vi "6229 Write_Rev1.vi"(0 "Arbitrary Waveform\nArray of Channels":T1(array[cluster])=[[{"AC Frequency (kHz)"=0.0, " Initial AC Ampl. (p-p/2)"=0.0, "Final AC Ampl."=0.0, "Initial DC Value"=7.0, "Final DC Value"=1.0, "Constant/Tau"=2.0, "Gamma AC"=1.0, "String"="Channel 0 A", "Gamma DC/Beta"=1.0}, {"AC Frequency (kHz)"=40.0, " Initial AC Ampl. (p-p/2)"=0.0, "Final AC Ampl."=0.0, "Initial DC Value"=1.0, "Final DC Value"=1.0, "Constant/Tau"=2.0, "Gamma AC"=1.0, "String"="Channel 0 B", "Gamma DC/Beta"=1.0}, {"AC Frequency (kHz)"=40.0, " Initial AC Ampl. (p-p/2)"=0.0, "Final AC Ampl."=0.0, "Initial DC Value"=1.0, "Final DC Value"=1.0, "Constant/Tau"=2.0, "Gamma AC"=1.0, "String"="Channel 0 C", "Gamma DC/Beta"=1.0}, {"AC Frequency (kHz)"=0.0, " Initial AC Ampl. (p-p/2)"=0.0, "Final AC Ampl."=0.0, "Initial DC Value"=1.0, "Final DC Value"=7.0, "Constant/Tau"=2.0, "Gamma AC"=0.0, "String"="Channel 0 D", "Gamma DC/Beta"=1.0}, {"AC Frequency (kHz)"=0.0, " Initial AC Ampl. (p-p/2)"=0.0, "Final AC Ampl."=0.0, "Initial DC Value"=7.0, "Final DC Value"=6.0, "Constant/Tau"=2.0, "Gamma AC"=0.0, "String"="Channel 0 E", "Gamma DC/Beta"=1.0}], [{"AC Frequency (kHz)"=10.0, " Initial AC Ampl. (p-p/2)"=5.0, "Final AC Ampl."=0.0, "Initial DC Value"=0.2, "Final DC Value"=0.16, "Constant/Tau"=0.25, "Gamma AC"=1.0, "String"="Channel 1 A", "Gamma DC/Beta"=1.0}, {"AC Frequency (kHz)"=10.0, " Initial AC Ampl. (p-p/2)"=5.0, "Final AC Ampl."=0.0, "Initial DC Value"=0.16, "Final DC Value"=0.16, "Constant/Tau"=0.25, "Gamma AC"=1.0, "String"="Channel 1 B", "Gamma DC/Beta"=1.0}, {"AC Frequency (kHz)"=10.0, " Initial AC Ampl. (p-p/2)"=0.0, "Final AC Ampl."=0.0, "Initial DC Value"=0.0, "Final DC Value"=0.0, "Constant/Tau"=0.25, "Gamma AC"=1.0, "String"="Channel 1 C", "Gamma DC/Beta"=1.0}, {"AC Frequency (kHz)"=0.0, " Initial AC Ampl. (p-p/2)"=0.0, "Final AC Ampl."=0.0, "Initial DC Value"=1.0, "Final DC Value"=1.0, "Constant/Tau"=199.2, "Gamma AC"=0.0, "String"="Channel 1 D", "Gamma DC/Beta"=1.0}, {"AC Frequency (kHz)"=0.0, " Initial AC Ampl. (p-p/2)"=0.0, "Final AC Ampl."=0.0, "Initial DC Value"=1.0, "Final DC Value"=1.0, "Constant/Tau"=199.2, "Gamma AC"=0.0, "String"="Channel 1 E", "Gamma DC/Beta"=1.0}], [{"AC Frequency (kHz)"=10.0, " Initial AC Ampl. (p-p/2)"=0.0, "Final AC Ampl."=0.0, "Initial DC Value"=0.007, "Final DC Value"=0.06, "Constant/Tau"=0.0, "Gamma AC"=1.0, "String"="Channel 2 A", "Gamma DC/Beta"=1.0}, {"AC Frequency (kHz)"=10.0, " Initial AC Ampl. (p-p/2)"=0.0, "Final AC Ampl."=0.0, "Initial DC Value"=0.06, "Final DC Value"=0.06, "Constant/Tau"=0.0, "Gamma AC"=1.0, "String"="Channel 2 B", "Gamma DC/Beta"=1.0}, {"AC Frequency (kHz)"=10.0, " Initial AC Ampl. (p-p/2)"=0.0, "Final AC Ampl."=0.0, "Initial DC Value"=0.0, "Final DC Value"=0.0, "Constant/Tau"=0.0, "Gamma AC"=1.0, "String"="Channel 2 C", "Gamma DC/Beta"=1.0}, {"AC Frequency (kHz)"=0.0, " Initial AC Ampl. (p-p/2)"=0.0, "Final AC Ampl."=0.0, "Initial DC Value"=1.0, "Final DC Value"=1.0, "Constant/Tau"=199.2, "Gamma AC"=0.0, "String"="", "Gamma DC/Beta"=1.0}, {"AC Frequency (kHz)"=0.0, " Initial AC Ampl. (p-p/2)"=0.0, "Final AC Ampl."=0.0, "Initial DC Value"=1.0, "Final DC Value"=1.0, "Constant/Tau"=199.2, "Gamma AC"=0.0, "String"="", "Gamma DC/Beta"=1.0}], [{"AC Frequency (kHz)"=10.0, " Initial AC Ampl. (p-p/2)"=0.0, "Final AC Ampl."=0.0, "Initial DC Value"=1.0, "Final DC Value"=1.0, "Constant/Tau"=199.2, "Gamma AC"=1.0, "String"="Channel 3 A", "Gamma DC/Beta"=1.0}, {"AC Frequency (kHz)"=10.0, " Initial AC Ampl. (p-p/2)"=0.0, "Final AC Ampl."=0.0, "Initial DC Value"=1.0, "Final DC Value"=1.0, "Constant/Tau"=199.2, "Gamma AC"=1.0, "String"="Channel 3 B", "Gamma DC/Beta"=1.0}, {"AC Frequency (kHz)"=10.0, " Initial AC Ampl. (p-p/2)"=0.0, "Final AC Ampl."=0.0, "Initial DC Value"=1.0, "Final DC Value"=1.0, "Constant/Tau"=199.2, "Gamma AC"=1.0, "String"="Channel 3 C", "Gamma DC/Beta"=1.0}, {"AC Frequency (kHz)"=0.0, " Initial AC Ampl. (p-p/2)"=0.0, "Final AC Ampl."=0.0, "Initial DC Value"=1.0, "Final DC Value"=1.0, "Constant/Tau"=199.2, "Gamma AC"=0.0, "String"="", "Gamma DC/Beta"=1.0}, {"AC Frequency (kHz)"=0.0, " Initial AC Ampl. (p-p/2)"=0.0, "Final AC Ampl."=0.0, "Initial DC Value"=1.0, "Final DC Value"=1.0, "Constant/Tau"=199.2, "Gamma AC"=0.0, "String"="", "Gamma DC/Beta"=1.0}], [{"AC Frequency (kHz)"=10.0, " Initial AC Ampl. (p-p/2)"=0.0, "Final AC Ampl."=0.0, "Initial DC Value"=-0.1, "Final DC Value"=-0.04, "Constant/Tau"=199.2, "Gamma AC"=1.0, "String"="Channel 4 A", "Gamma DC/Beta"=1.0}, {"AC Frequency (kHz)"=10.0, " Initial AC Ampl. (p-p/2)"=0.0, "Final AC Ampl."=0.0, "Initial DC Value"=-0.1, "Final DC Value"=-0.04, "Constant/Tau"=199.2, "Gamma AC"=1.0, "String"="Channel 4 B", "Gamma DC/Beta"=1.0}, {"AC Frequency (kHz)"=10.0, " Initial AC Ampl. (p-p/2)"=0.0, "Final AC Ampl."=0.0, "Initial DC Value"=-0.1, "Final DC Value"=-0.04, "Constant/Tau"=199.2, "Gamma AC"=1.0, "String"="Channel 4 C", "Gamma DC/Beta"=1.0}, {"AC Frequency (kHz)"=0.0, " Initial AC Ampl. (p-p/2)"=0.0, "Final AC Ampl."=0.0, "Initial DC Value"=1.0, "Final DC Value"=1.0, "Constant/Tau"=199.2, "Gamma AC"=0.0, "String"="", "Gamma DC/Beta"=1.0}, {"AC Frequency (kHz)"=0.0, " Initial AC Ampl. (p-p/2)"=0.0, "Final AC Ampl."=0.0, "Initial DC Value"=1.0, "Final DC Value"=1.0, "Constant/Tau"=199.2, "Gamma AC"=0.0, "String"="", "Gamma DC/Beta"=1.0}], [{"AC Frequency (kHz)"=10.0, " Initial AC Ampl. (p-p/2)"=0.0, "Final AC Ampl."=0.0, "Initial DC Value"=-0.1, "Final DC Value"=-0.04, "Constant/Tau"=199.2, "Gamma AC"=1.0, "String"="Channel 5 A", "Gamma DC/Beta"=1.0}, {"AC Frequency (kHz)"=10.0, " Initial AC Ampl. (p-p/2)"=0.0, "Final AC Ampl."=0.0, "Initial DC Value"=-0.1, "Final DC Value"=-0.04, "Constant/Tau"=199.2, "Gamma AC"=1.0, "String"="Channel 5 B", "Gamma DC/Beta"=1.0}, {"AC Frequency (kHz)"=10.0, " Initial AC Ampl. (p-p/2)"=0.0, "Final AC Ampl."=0.0, "Initial DC Value"=-0.1, "Final DC Value"=-0.04, "Constant/Tau"=199.2, "Gamma AC"=1.0, "String"="Channel 5 C", "Gamma DC/Beta"=1.0}, {"AC Frequency (kHz)"=0.0, " Initial AC Ampl. (p-p/2)"=0.0, "Final AC Ampl."=0.0, "Initial DC Value"=1.0, "Final DC Value"=1.0, "Constant/Tau"=199.2, "Gamma AC"=0.0, "String"="", "Gamma DC/Beta"=1.0}, {"AC Frequency (kHz)"=0.0, " Initial AC Ampl. (p-p/2)"=0.0, "Final AC Ampl."=0.0, "Initial DC Value"=1.0, "Final DC Value"=1.0, "Constant/Tau"=199.2, "Gamma AC"=0.0, "String"="", "Gamma DC/Beta"=1.0}], [{"AC Frequency (kHz)"=10.0, " Initial AC Ampl. (p-p/2)"=0.0, "Final AC Ampl."=0.0, "Initial DC Value"=-0.1, "Final DC Value"=-0.04, "Constant/Tau"=199.2, "Gamma AC"=1.0, "String"="Channel 6 A", "Gamma DC/Beta"=1.0}, {"AC Frequency (kHz)"=10.0, " Initial AC Ampl. (p-p/2)"=0.0, "Final AC Ampl."=0.0, "Initial DC Value"=-0.1, "Final DC Value"=-0.04, "Constant/Tau"=199.2, "Gamma AC"=1.0, "String"="Channel 6 B", "Gamma DC/Beta"=1.0}, {"AC Frequency (kHz)"=10.0, " Initial AC Ampl. (p-p/2)"=0.0, "Final AC Ampl."=0.0, "Initial DC Value"=-0.1, "Final DC Value"=-0.04, "Constant/Tau"=199.2, "Gamma AC"=1.0, "String"="Channel 6 C", "Gamma DC/Beta"=1.0}, {"AC Frequency (kHz)"=0.0, " Initial AC Ampl. (p-p/2)"=0.0, "Final AC Ampl."=0.0, "Initial DC Value"=1.0, "Final DC Value"=1.0, "Constant/Tau"=199.2, "Gamma AC"=0.0, "String"="", "Gamma DC/Beta"=1.0}, {"AC Frequency (kHz)"=0.0, " Initial AC Ampl. (p-p/2)"=0.0, "Final AC Ampl."=0.0, "Initial DC Value"=1.0, "Final DC Value"=1.0, "Constant/Tau"=199.2, "Gamma AC"=0.0, "String"="", "Gamma DC/Beta"=1.0}], [{"AC Frequency (kHz)"=10.0, " Initial AC Ampl. (p-p/2)"=0.0, "Final AC Ampl."=0.0, "Initial DC Value"=-0.1, "Final DC Value"=-0.04, "Constant/Tau"=199.2, "Gamma AC"=1.0, "String"="Channel 7 A", "Gamma DC/Beta"=1.0}, {"AC Frequency (kHz)"=10.0, " Initial AC Ampl. (p-p/2)"=0.0, "Final AC Ampl."=0.0, "Initial DC Value"=-0.1, "Final DC Value"=-0.04, "Constant/Tau"=199.2, "Gamma AC"=1.0, "String"="Channel 7 B", "Gamma DC/Beta"=1.0}, {"AC Frequency (kHz)"=10.0, " Initial AC Ampl. (p-p/2)"=0.0, "Final AC Ampl."=0.0, "Initial DC Value"=-0.1, "Final DC Value"=-0.04, "Constant/Tau"=199.2, "Gamma AC"=1.0, "String"="Channel 7 C", "Gamma DC/Beta"=1.0}, {"AC Frequency (kHz)"=0.0, " Initial AC Ampl. (p-p/2)"=0.0, "Final AC Ampl."=0.0, "Initial DC Value"=1.0, "Final DC Value"=1.0, "Constant/Tau"=199.2, "Gamma AC"=0.0, "String"="", "Gamma DC/Beta"=1.0}, {"AC Frequency (kHz)"=0.0, " Initial AC Ampl. (p-p/2)"=0.0, "Final AC Ampl."=0.0, "Initial DC Value"=1.0, "Final DC Value"=1.0, "Constant/Tau"=199.2, "Gamma AC"=0.0, "String"="", "Gamma DC/Beta"=1.0}]] {"Gamma DC/Beta" format="%.2f"; "Gamma AC" format="%.2f"; "Constant/Tau" min=0.0 max=240.0 format="%.4f"; "Final DC Value" format="%.3f"; "Initial DC Value" format="%.3f"; "Final AC Ampl." format="%.3f"; "Initial AC Ampl. (p-p/2)" format="%.3f"; "AC Frequency (kHz)" format="%.2f"}, 2 "Channel to plot":i32 min=0 max=7, 3 "Unit Conversions":u16[](array[ring])=[0, 0, 2, 3, 4, 0, 0, 0] items=["Volts-to-Volts Power Law", "Evaporation Formula", "Dimple Evaporation"], 4 "Interval Lengths (ms)":dbl[](array[numeric])=[120.0, 16.0, 484.0, 700.0, 100.0] format="%.3f", 5 "Channel Controls":bool[](array[boolean])=[TRUE, TRUE, FALSE, FALSE, FALSE, FALSE, FALSE, FALSE], 6 "ON or OFF?":bool[](array[boolean])=[TRUE, TRUE, TRUE, FALSE, FALSE], 11 "error in":errorcluster, 12 "Dither Control":u16(ring)=1 items=["Disable Dither", "Enable Dither"]) -> (9 "Sampling Rate":dbl=2882.3529411764707 format="%.2f", 10 "= Total Waveform\nTime (ms)":dbl=1420.0 format="%.3f", 13 "Waveform on Channel to Plot":cluster{dbl[], dbl[]}(graph), 14 "signal out":waveform(dbl)[](graph)=[{"t0"=timestamp(0 s since 1904-01-01), "dt"=0.00034693877551020405, "Y"=array[4091 elements]}, {"t0"=timestamp(0 s since 1904-01-01), "dt"=0.00034693877551020405, "Y"=array[4091 elements]}], 15 "error out":errorcluster)   [LabVIEW 2013]
uses:
  <vilib>/Utility/error.llb/DialogType.ctl
  <vilib>/DAQmx/write.llb/DAQmx Write (Analog 1D Wfm NChan NSamp).vi
  <vilib>/DAQmx/configure/timing.llb/DAQmx Timing (Sample Clock).vi
  <vilib>/DAQmx/create/channels.llb/DAQmx Create Channel (CO-Pulse Generation-Frequency).vi
  <vilib>/DAQmx/configure/timing.llb/DAQmx Timing (Implicit).vi
  <vilib>/DAQmx/configure/trigger.llb/DAQmx Start Trigger (Digital Edge).vi
  <vilib>/DAQmx/miscellaneous.llb/DAQmx Fill In Error Info.vi
  <resource>/objmgr/daqmx.rc
panel:
  in  "Case Constant\n(See Context Help) 3":bool=TRUE
  in  "Case Constant\n(See Context Help) 2":bool
  in  "Dither Control":u16
  in  "Case Constant\n(See Context Help)":bool
  in  "Dither Control":u16
  out "number of samples written per channel":u32
  out "Pmod Graph":dbl[][](graph)
  out "wvfrm size":i32=4091
  out "x+y 2":dbl=1.42
  out "Numeric":i32=287
  out "6229 counter task out":refnum<k21>="Counter Output"
  out "6229 lattice loading task out":refnum<k21>="Adiabatic Loading"
  out "Array":dbl[][](array[numeric])
  out "6229 Status":string="PCI-6221 OK"
  out "total points":dbl=4092.0 format="%.2f"
  out "Points per Segment":dbl[](array[numeric])=[345.0, 46.0, 1395.0, 2017.0, 288.0] format="%.2f"
  # "Warning! Constant for interval A does not set all intervals for 86 Sr frequency"
  # "Controls"
  # "Volts to Volts Power Law Formula\nf100=DCinitial +(DCfinal-DCinitial)*(time/intervaltime)**gammaDC;"
  # "Don't change"
  # "Note: B-field to Voltage\nConversion not yet\nimplemented.  Must \ninsert appropriate\nformulae."
  # "CH 0"
  # "CH 1"
  # "CH 2"
  # "CH 3"
  # "Evaporation Formula\nf100=Initial/((1+(time/tau))**beta)+Final;"
  # "Initial DC = U1, Constant = Tau\nGamma DC = Beta"
  # "Interval A"
  # "Interval B"
  # "Interval C"
  # "Interval D"
  # "Interval E"
  # "Interval F"
  # "Output"
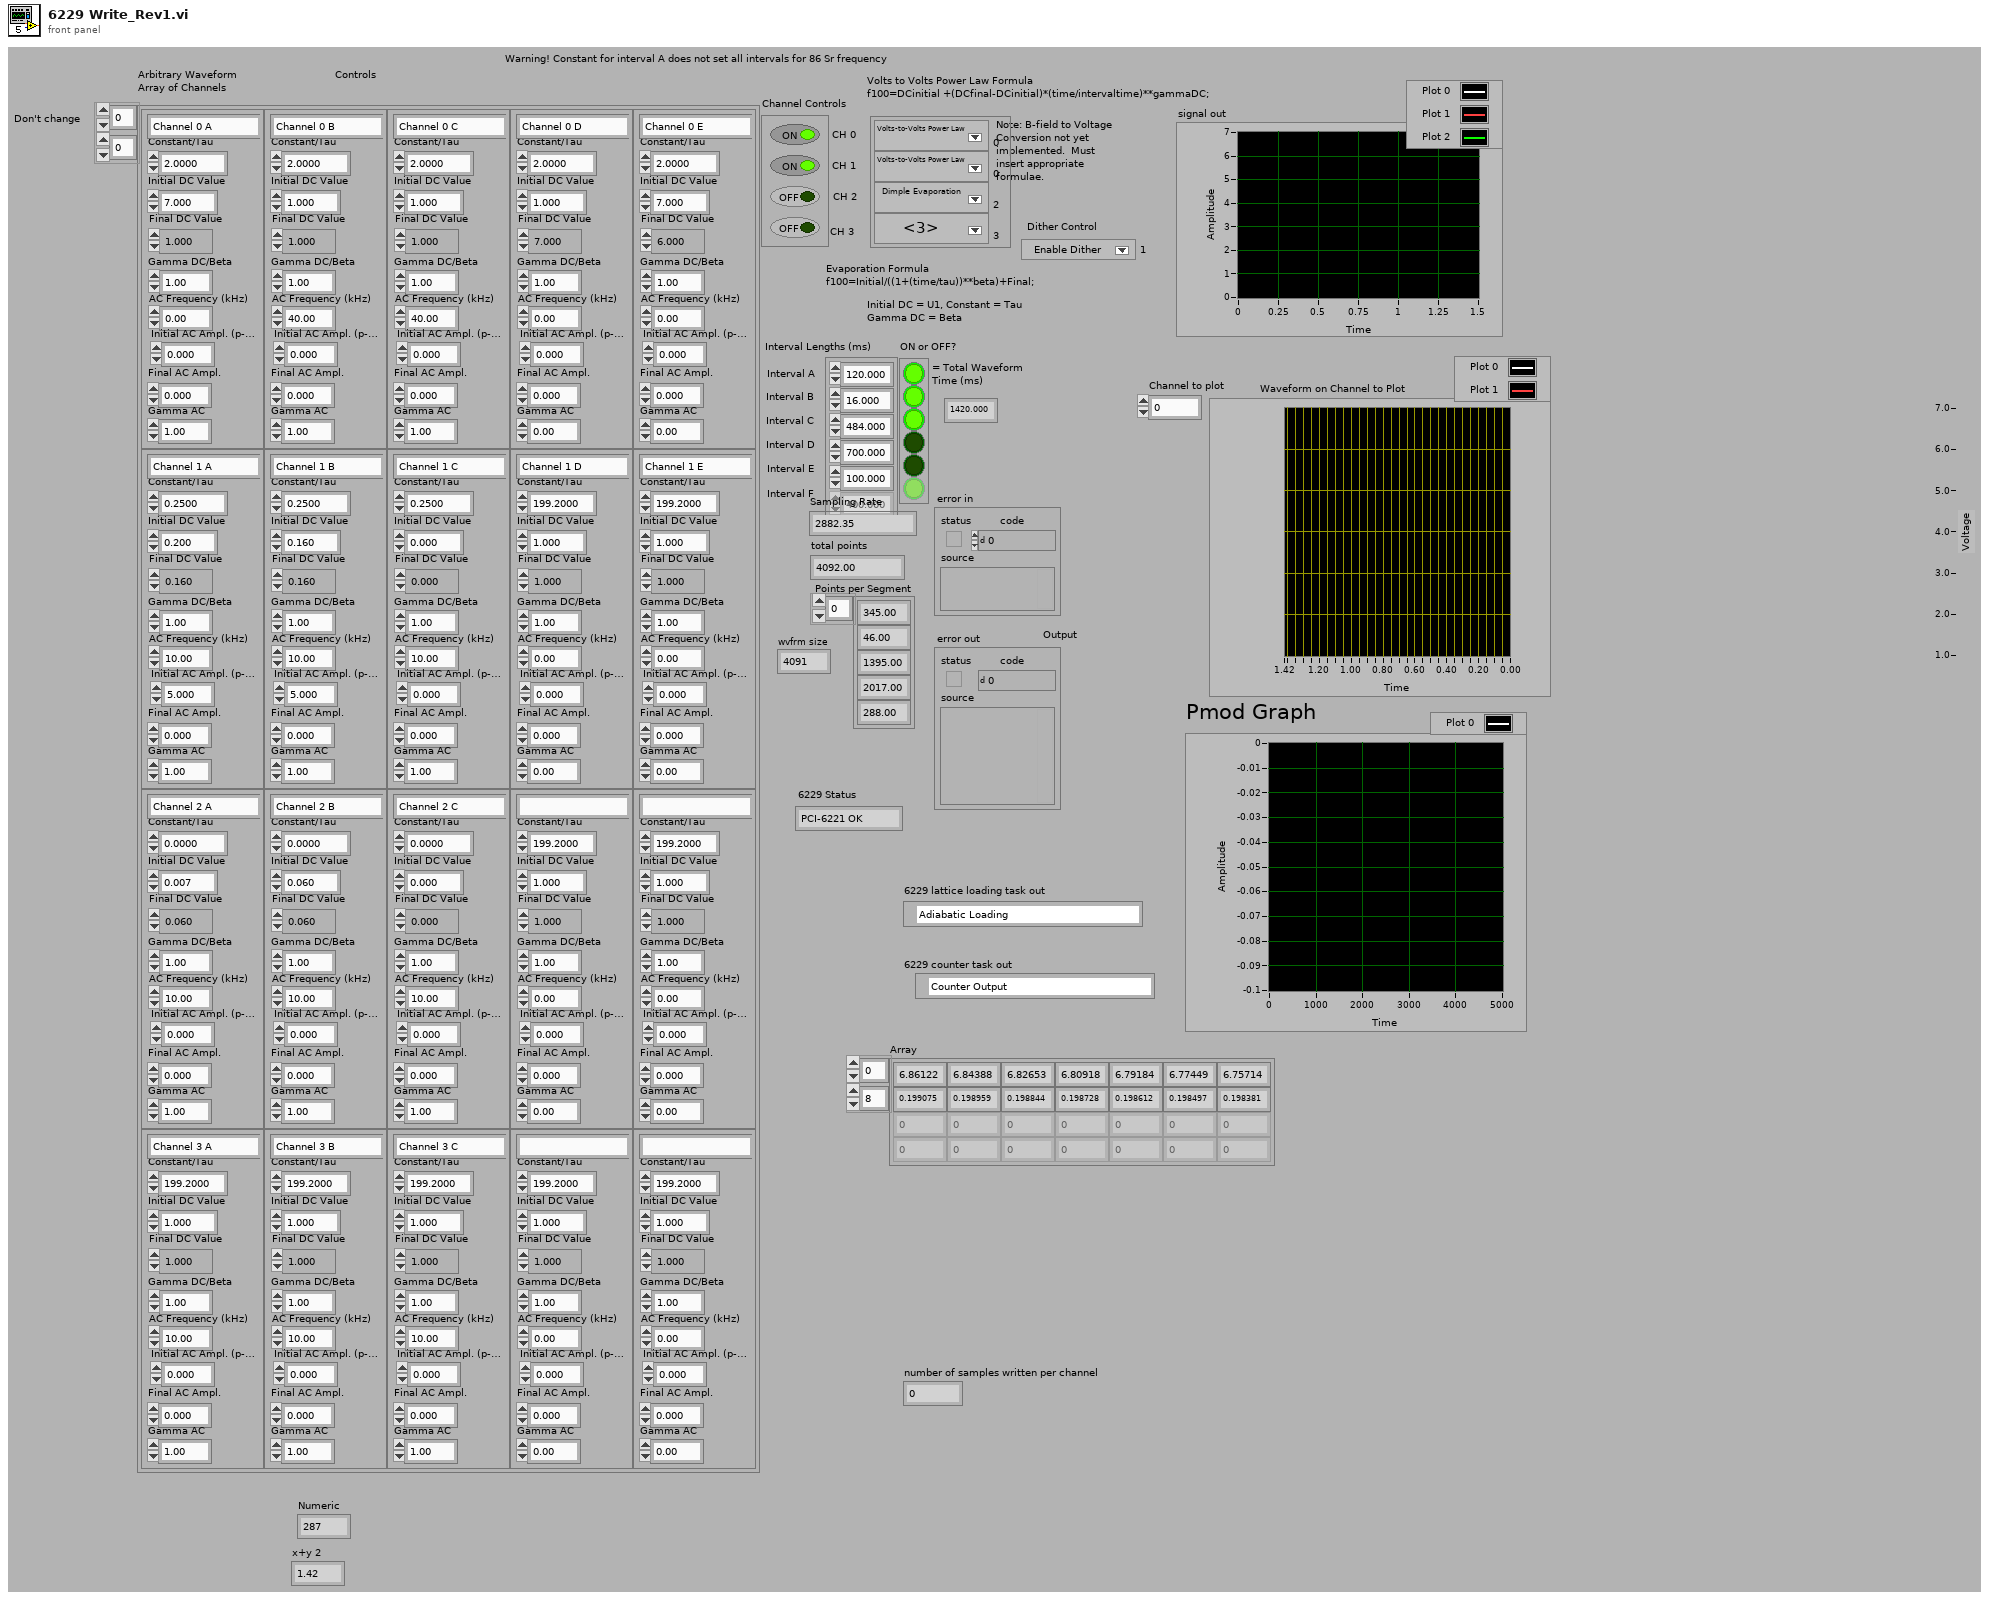
[diagram p1: front panel]
types:
  T1 = cluster{"AC Frequency (kHz)":dbl, " Initial AC Ampl. (p-p/2)":dbl, "Final AC Ampl.":dbl, "Initial DC Value":dbl, "Final DC Value":dbl, "Constant/Tau":dbl, "Gamma AC":dbl, "String":string, "Gamma DC/Beta":dbl}[][]
  T2 = cluster{"AC Frequency (kHz)":dbl, " Initial AC Ampl. (p-p/2)":dbl, "Final AC Ampl.":dbl, "Initial DC Value":dbl, "Final DC Value":dbl, "Constant/Tau":dbl, "Gamma AC":dbl, "String":string, "Gamma DC/Beta":dbl}
  T3 = cluster{"AC Frequency (kHz)":dbl, " Initial AC Ampl. (p-p/2)":dbl, "Final AC Ampl.":dbl, "Initial DC Value":dbl, "Final DC Value":dbl, "Constant/Tau":dbl, "Gamma AC":dbl, "String":string, "Gamma DC/Beta":dbl}[]
  T4 = typedef "DialogType.ctl" = u16
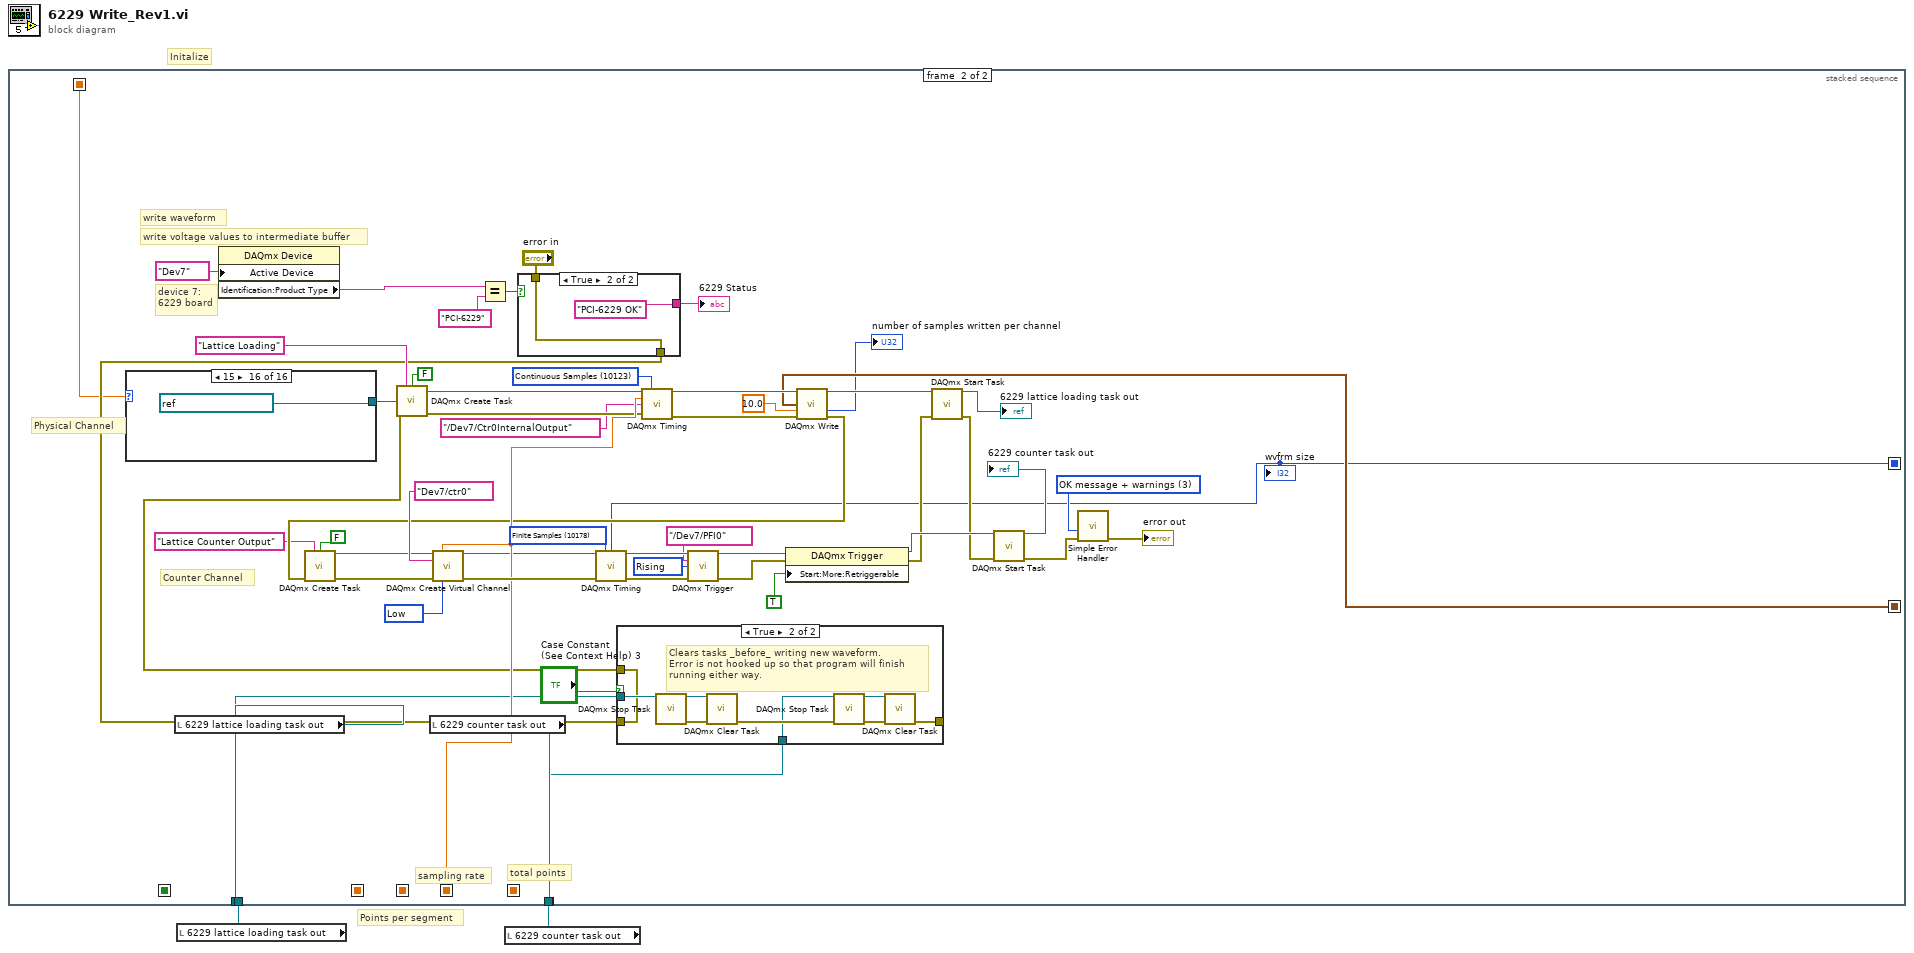
[diagram p0: block diagram]
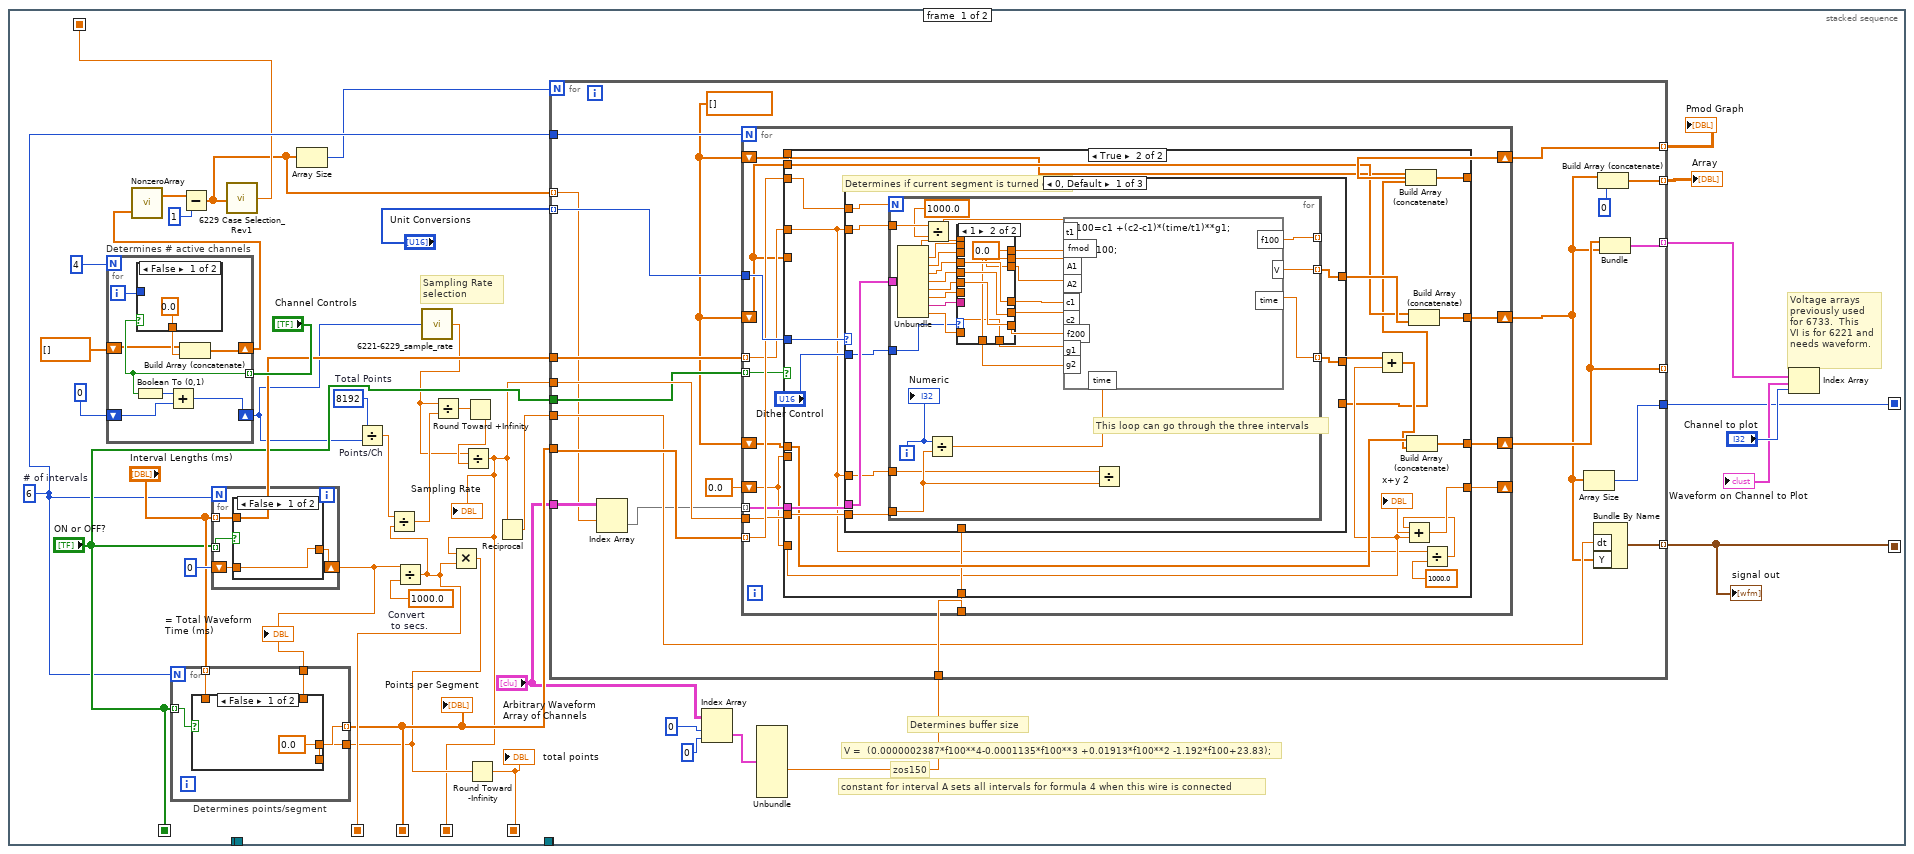
[diagram p2: hidden frame]
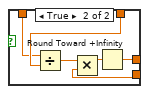
[diagram p3: hidden frame]
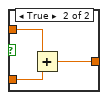
[diagram p4: hidden frame]
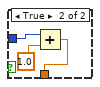
[diagram p5: hidden frame]
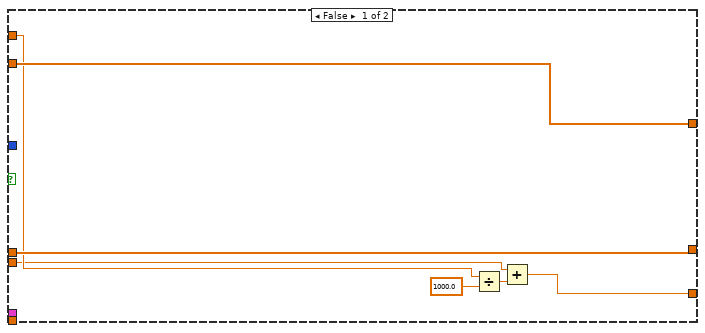
[diagram p6: hidden frame]
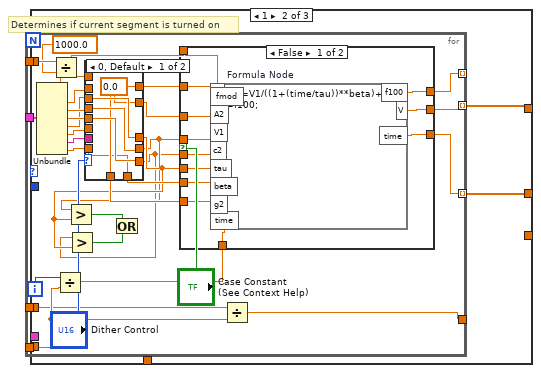
[diagram p8: hidden frame]
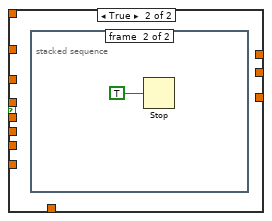
[diagram p9: hidden frame]
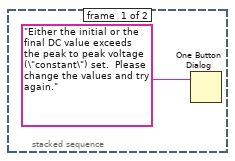
[diagram p10: hidden frame]
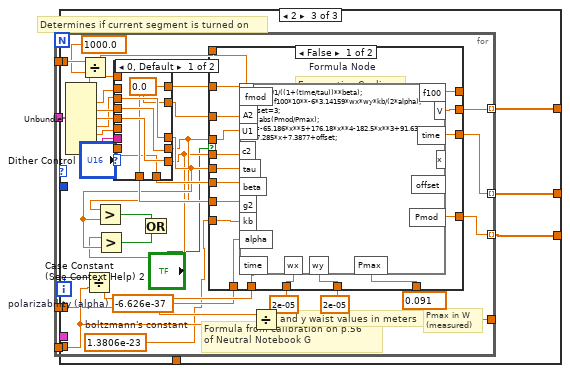
[diagram p12: hidden frame]
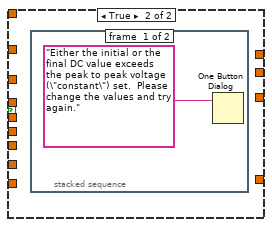
[diagram p13: hidden frame]
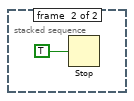
[diagram p14: hidden frame]
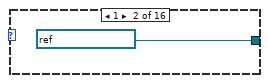
[diagram p17: hidden frame]
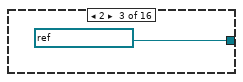
[diagram p18: hidden frame]
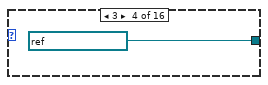
[diagram p19: hidden frame]
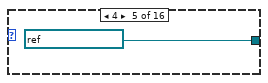
[diagram p20: hidden frame]
diagram:
  # "Points per segment"
  # "Initalize"
  n1 = local read "6229 lattice loading task out"() -> (w3:refnum<k21>)
  n2 = local read "6229 lattice loading task out"() -> (w2:refnum<k21>)
  n3 = local read "6229 counter task out"() -> (w4:refnum<k21>)
  n4 = local read "6229 counter task out"() -> (w1:refnum<k21>)
  n5 = stacked-sequence {
    seq-local: [w21 _] -> [_ w361]
    seq-local: [w32 _] -> [_ _]
    seq-local: ["ON or OFF?" _] -> [_ _]
    seq-local: [w7 _] -> [_ _]
    seq-local: [w34 _] -> [_ _]
    seq-local: [w19 _] -> [_ w335]
    seq-local: [w11 _] -> [_ w336]
    seq-local: [w18 _] -> [_ w334]
    tunnel: w3 -> [_ w346]
    tunnel: w4 -> [_ w347]
    tunnel: w2 -> [_ _]
    tunnel: w1 -> [_ _]
    frame #0 {
      w17 = 6  # # of intervals
      w46 = 8192  # Total Points
      # "Sampling Rate selection"
      # "Voltage arrays\npreviously used\nfor 6733.  This\nVI is for 6221 and\nneeds waveform."
      # "zos150"
      # "Determines buffer size"
      # "constant for interval A sets all intervals for formula 4 when this wire is connected"
      # "V =  (0.0000002387*f100**4-0.0001135*f100**3 +0.01913*f100**2 -1.192*f100+23.83);"
      n6 = for "Determines # active channels" {
        N: 4 -> [_]
        tunnel: "Channel Controls" -> [w71] mode=indexing
        shift-right: [w72] -> w6
        shift-left: 0 -> [w73]
        shift-right: [w69] -> w14
        shift-left: dbl[] [] -> [w67]
        i -> [w70]
        n7 = Boolean To (0,1)(Boolean=w71) -> (0, 1=w74:i16)
        n8 = case shown="False" w71 {
          tunnel: w70 -> [_ w77]
          tunnel: [0.0 w76] -> w68
          frame False {
          }
          frame True {
            n9 = Add(x=w77, y=1.0) -> (x+y=w76:dbl)
          }
        }
        n10 = Add(x=w74, y=w73) -> (x+y=w72:i32)
        n11 = Build Array (concatenate)(w67, w68) -> (w69:dbl[])
      }
      n12 = call "NonzeroArray.vi"("Input Array"=w14) -> ("Output Array"=w13:dbl[])
      n13 = Subtract(x=w13, y=1) -> (x-y=w8:dbl[])
      n14 = for {
        N: w17 -> [_]
        tunnel: "Interval Lengths (ms)" -> [w60] mode=indexing
        tunnel: "ON or OFF?" -> [w62] mode=indexing
        shift-right: [w59] -> w35
        shift-left: 0 -> [w61]
        n15 = case shown="False" w62 {
          tunnel: w61 -> [w63 w66]
          tunnel: w60 -> [_ w65]
          tunnel: [w63 w64] -> w59
          frame False {
          }
          frame True {
            n16 = Add(x=w65, y=w66) -> (x+y=w64:dbl)
          }
        }
      }
      "= Total Waveform\nTime (ms)" <- w35
      n17 = call "6229 Case Selection_Rev1.vi"("Input Array"=w8) -> ("DAQ Channel Case"=w11:dbl)
      n18 = Array Size(array=w8) -> (size(s)=w9:i32)
      n19 = Divide "Points/Ch"(x=w46, y=w6) -> (x/y=w33:dbl)
      n20 = Divide "Convert\n to secs."(x=w35, y=1000.0) -> (x/y=w34:dbl)
      n21 = Divide(x=w33, y=w34) -> (x/y=w40:dbl)
      n22 = call "6221-6229_sample_rate.vi"("# of output channels"=w6) -> ("Sampling rate"=w5:dbl)
      n23 = Divide(x=w5, y=w40) -> (x/y=w39:dbl)
      n24 = Round Toward +Infinity(x=w39) -> (ceil(x): smallest int >= x=w38:dbl)
      n25 = Divide(x=w5, y=w38) -> (x/y=w21:dbl)
      "Sampling Rate" <- w21
      n26 = Multiply(x=w21, y=w34) -> (x*y=w30:dbl)
      n27 = for "Determines points/segment" {
        N: w17 -> [_]
        tunnel: "ON or OFF?" -> [w51] mode=indexing
        tunnel: "Interval Lengths (ms)" -> [w50] mode=indexing
        tunnel: w35 -> [w49]
        tunnel: [w48] -> w32 mode=indexing
        tunnel: w30 -> [w47]
        n28 = case shown="False" w51 {
          tunnel: w50 -> [_ w57]
          tunnel: w49 -> [_ w58]
          tunnel: [0.0 w54] -> w48
          tunnel: w47 -> [_ w55]
          frame False {
          }
          frame True {
            n29 = Divide(x=w57, y=w58) -> (x/y=w56:dbl)
            n30 = Multiply(x=w56, y=w55) -> (x*y=w53:dbl)
            n31 = Round Toward +Infinity(x=w53) -> (ceil(x): smallest int >= x=w54:dbl)
          }
        }
      }
      "Points per Segment" <- w32
      n32 = Round Toward -Infinity(1:w30) -> (0:w7:dbl)
      "total points" <- w7
      n33 = Reciprocal(x=w21) -> (1/x=w20:dbl)
      n34 = Index Array(array="Arbitrary Waveform\nArray of Channels", index (row)=0, index (col)=0 ("disabled index (col)")) -> (element=w25:T2)
      n35 = Unbundle(w25) -> ("Constant/Tau"=w24:dbl)  [unwired: 8 out]
      n36 = for {
        N: w9 -> [_]
        tunnel: "Unit Conversions" -> [w99] mode=indexing
        tunnel: "Arbitrary Waveform\nArray of Channels" -> [w81]
        tunnel: w32 -> [w98]
        tunnel: w21 -> [w97]
        tunnel: "Interval Lengths (ms)" -> [w96]
        tunnel: "ON or OFF?" -> [w95]
        tunnel: [w88] -> _ mode=indexing
        tunnel: [w92] -> w29 mode=indexing
        tunnel: [w94] -> w36 mode=indexing
        tunnel: w24 -> [w91]
        tunnel: w20 -> [w90]
        tunnel: [w89] -> w19 mode=indexing
        tunnel: [w86] -> w18
        tunnel: w17 -> [w85]
        tunnel: [w84] -> w16 mode=indexing
        tunnel: w8 -> [w80] mode=indexing
        w82 = dbl[] []
        n37 = Index Array(array=w81, index (row)=w80) -> (element=w79:T3)  [unwired: 1 in]
        n38 = for {
          N: w85 -> [_]
          tunnel: w79 -> [w112] mode=indexing
          tunnel: w99 -> [w114]
          tunnel: w98 -> [w113] mode=indexing
          tunnel: w97 -> [w111]
          tunnel: w96 -> [w110] mode=indexing
          tunnel: w95 -> [w109] mode=indexing
          shift-right: [w103] -> w88
          shift-left: w82 -> [w108]
          shift-right: [w107] -> _
          shift-left: 0.0 -> [w102]
          shift-right: [w106] -> w87
          shift-left: w82 -> [w105]
          tunnel: w91 -> [w104]
          shift-right: [w100] -> w84
          shift-left: w82 -> [w101]
          n39 = case shown="True" w109 {
            tunnel: w114 -> [_ w135]
            tunnel: w113 -> [_ w131]
            tunnel: w112 -> [_ w142]
            tunnel: w111 -> [_ w141]
            tunnel: w110 -> [w117 w125]
            tunnel: [w121 w140] -> w103
            tunnel: w108 -> [w121 w139]
            tunnel: [w116 w132] -> w107
            tunnel: [w120 w138] -> w106
            tunnel: w105 -> [_ w136]
            tunnel: w105 -> [w120 _]
            tunnel: w104 -> [_ w133]
            tunnel: w102 -> [_ w126]
            tunnel: w102 -> [w115 _]
            tunnel: [_ w123] -> w100
            tunnel: w101 -> [_ w122]
            frame False {
              n40 = Divide(x=w117, y=1000.0) -> (x/y=w119:dbl)
              n41 = Add(x=w115, y=w119) -> (x+y=w116:dbl)
            }
            frame True {
              # "Determines if current segment is turned on"
              n42 = case shown="0, Default" w135 {
                tunnel: w131 -> [w150 w199 w264]
                tunnel: w142 -> [w149 w198 w263]
                tunnel: w141 -> [w145 w194 w259]
                tunnel: w125 -> [w148 w197 w262]
                tunnel: [w147 w196 w261] -> w137
                tunnel: [w146 w195 w260] -> w128
                tunnel: w125 -> [w144 w193 w258]
                tunnel: "Dither Control" -> [w143 _ _]
                tunnel: w133 -> [_ _ _]
                tunnel: [_ _ w257] -> w124
                frame 0, Default {
                  n43 = for {
                    N: w150 -> [_]
                    tunnel: w149 -> [w179]
                    tunnel: w145 -> [w158]
                    tunnel: w148 -> [w178]
                    tunnel: [w151] -> w147 mode=indexing
                    tunnel: [w157] -> w146 mode=indexing
                    tunnel: [w156] -> _ mode=indexing
                    tunnel: w144 -> [w154]
                    tunnel: w143 -> [w155]
                    i -> [w176]
                    # "Volts-to-Volts Power Law"
                    # "This loop can go through the three intervals"
                    n44 = Unbundle(w179) -> ("AC Frequency (kHz)"=w172:dbl, "Initial AC Ampl. (p-p/2)"=w171:dbl, "Final AC Ampl."=w170:dbl, "Initial DC Value"=w152:dbl, "Final DC Value"=w169:dbl, "Constant/Tau"=w173:dbl, "Gamma AC"=w174:dbl, "String"=w175:string, "Gamma DC/Beta"=w160:dbl)
                    n45 = Divide(x=w178, y=1000.0) -> (x/y=w168:dbl)
                    n46 = Divide(x=w176, y=w158) -> (x/y=w153:dbl)
                    n47 = case shown="1" w155 {
                      tunnel: w175 -> [_ _]
                      tunnel: w174 -> [w181 _]
                      tunnel: w173 -> [w182 w190]
                      tunnel: w172 -> [w187 _]
                      tunnel: w171 -> [w186 _]
                      tunnel: w170 -> [w185 _]
                      tunnel: w152 -> [w184 w192]
                      tunnel: w169 -> [w183 w191]
                      tunnel: [w187 w189] -> w167
                      tunnel: [w186 w189] -> w166
                      tunnel: [w185 w189] -> w165
                      tunnel: [w184 w192] -> w164
                      tunnel: [w183 w191] -> w163
                      tunnel: [w182 w190] -> w162
                      tunnel: [w181 w189] -> w161
                      tunnel: w160 -> [w180 w188]
                      tunnel: [w180 w188] -> w159
                      frame 0, Default {
                      }
                      frame 1 {
                        w189 = 0.0 ("AC Frequency (kHz)")
                      }
                    }
                    n48 = formula code="f100=c1 +(c2-c1)*(time/t1)**g1;\n\nV = f100;"("c1"=w164, "time"=w153, "t1"=w168, "c2"=w163, "f200"=w162, "fmod"=w167, "A1"=w166, "A2"=w165, "g1"=w159, "g2"=w161) -> ("f100"=w156:dbl, "time"=w157:dbl, "V"=w151:dbl)
                    n49 = Divide(x=w154, y=w158) -> ()  [unwired: 1 out]
                    "Numeric" <- w176
                  }
                }
                frame 1 {
                  # "Determines if current segment is turned on"
                  n50 = for {
                    N: w199 -> [_]
                    tunnel: w198 -> [w230]
                    tunnel: w194 -> [w214]
                    tunnel: w197 -> [w226]
                    tunnel: [w229] -> w196 mode=indexing
                    tunnel: [w228] -> w195 mode=indexing
                    tunnel: [w227] -> _ mode=indexing
                    tunnel: [w213] -> _
                    tunnel: w193 -> [w201]
                    i -> [w224]
                    n51 = Unbundle(w230) -> ("AC Frequency (kHz)"=w207:dbl, "Final AC Ampl."=w208:dbl, "Initial DC Value"=w211:dbl, "Final DC Value"=w210:dbl, "Constant/Tau"=w209:dbl, "Gamma AC"=w222:dbl, "String"=w223:string, "Gamma DC/Beta"=w217:dbl)  [unwired: 1 out]
                    n52 = Divide(x=w226, y=1000.0) -> (x/y=w221:dbl)
                    n53 = Divide(x=w224, y=w214) -> (x/y=w215:dbl)
                    n54 = case shown="0, Default" "Dither Control" {
                      tunnel: w223 -> [_ _]
                      tunnel: w222 -> [_ w252]
                      tunnel: w210 -> [w247 w253]
                      tunnel: w208 -> [_ w256]
                      tunnel: w209 -> [w249 w255]
                      tunnel: w211 -> [w248 w254]
                      tunnel: [w246 w250] -> w220
                      tunnel: [w246 w256] -> w219
                      tunnel: [w249 w255] -> w204
                      tunnel: [w248 w254] -> w203
                      tunnel: [w247 w253] -> w202
                      tunnel: [w246 w252] -> w218
                      tunnel: w217 -> [w245 w251]
                      tunnel: [w245 w251] -> w216
                      tunnel: w207 -> [_ w250]
                      frame 0, Default {
                        w246 = 0.0 ("AC Frequency (kHz)")
                      }
                      frame 1 {
                      }
                    }
                    n55 = Greater?(x=w203, y=w204) -> (0:w205:bool)
                    n56 = Greater?(x=w202, y=w204) -> (0:w206:bool)
                    n57 = Or(x=w205, y=w206) -> ()  [unwired: 1 out]
                    n58 = case shown="False" "Case Constant\n(See Context Help)" {
                      tunnel: [w242 _] -> w229
                      tunnel: [w241 _] -> w228
                      tunnel: [w240 _] -> w227
                      tunnel: w221 -> [w239 _]
                      tunnel: w220 -> [w238 _]
                      tunnel: w219 -> [w237 _]
                      tunnel: w218 -> [w236 _]
                      tunnel: w216 -> [w235 _]
                      tunnel: w215 -> [w234 _]
                      tunnel: w203 -> [w233 _]
                      tunnel: w202 -> [w232 _]
                      tunnel: w204 -> [w231 _]
                      frame False {
                        # "Evaporative Cooling"
                        n59 = formula code="f100=V1/((1+(time/tau))**beta)+c2;\nV=f100;"("V1"=w233, "time"=w234, "t1"=w239, "c2"=w232, "tau"=w231, "fmod"=w238, "A2"=w237, "beta"=w235, "g2"=w236) -> ("f100"=w240:dbl, "time"=w241:dbl, "V"=w242:dbl)
                      }
                      frame True {
                        n60 = stacked-sequence {
                          frame #0 {
                            n61 = One Button Dialog(message="Either the initial or the final DC value exceeds the peak to peak voltage (\"constant\") set.  Please change the values and try again.") -> ()  [unwired: 1 in, 1 out]
                          }
                          frame #1 {
                            n62 = Stop(stop? (T)=TRUE) -> ()
                          }
                        }
                      }
                    }
                    n63 = Divide(x=w201, y=w214) -> (x/y=w213:dbl)
                  }
                }
                frame 2 {
                  # "Determines if current segment is turned on"
                  n64 = for {
                    N: w264 -> [_]
                    tunnel: w263 -> [w300]
                    tunnel: w259 -> [w285]
                    tunnel: w262 -> [w297]
                    tunnel: [w299] -> w261 mode=indexing
                    tunnel: [w298] -> w260 mode=indexing
                    tunnel: [w284] -> _
                    tunnel: w258 -> [w272]
                    tunnel: [w265] -> w257 mode=indexing
                    i -> [w295]
                    w270 = -6.626e-37  # polarizability (alpha)
                    w269 = 1.3806e-23  # boltzmann's constant
                    # "Pmax in W\n(measured)"
                    # "x and y waist values in meters"
                    # "Formula from calibration on p.56 \nof Neutral Notebook G"
                    n65 = Unbundle(w300) -> ("AC Frequency (kHz)"=w278:dbl, "Final AC Ampl."=w279:dbl, "Initial DC Value"=w282:dbl, "Final DC Value"=w281:dbl, "Constant/Tau"=w280:dbl, "Gamma AC"=w293:dbl, "String"=w294:string, "Gamma DC/Beta"=w288:dbl)  [unwired: 1 out]
                    n66 = Divide(x=w297, y=1000.0) -> (x/y=w292:dbl)
                    n67 = Divide(x=w295, y=w285) -> (x/y=w286:dbl)
                    n68 = case shown="0, Default" "Dither Control" {
                      tunnel: w294 -> [_ _]
                      tunnel: w293 -> [_ w328]
                      tunnel: w281 -> [w323 w329]
                      tunnel: w279 -> [_ w332]
                      tunnel: w280 -> [w325 w331]
                      tunnel: w282 -> [w324 w330]
                      tunnel: [w322 w326] -> w291
                      tunnel: [w322 w332] -> w290
                      tunnel: [w325 w331] -> w275
                      tunnel: [w324 w330] -> w274
                      tunnel: [w323 w329] -> w273
                      tunnel: [w322 w328] -> w289
                      tunnel: w288 -> [w321 w327]
                      tunnel: [w321 w327] -> w287
                      tunnel: w278 -> [_ w326]
                      frame 0, Default {
                        w322 = 0.0 ("AC Frequency (kHz)")
                      }
                      frame 1 {
                      }
                    }
                    n69 = Greater?(x=w274, y=w275) -> (0:w276:bool)
                    n70 = Greater?(x=w273, y=w275) -> (0:w277:bool)
                    n71 = Or(x=w276, y=w277) -> ()  [unwired: 1 out]
                    n72 = case shown="False" "Case Constant\n(See Context Help) 2" {
                      tunnel: [w318 _] -> w299
                      tunnel: [w317 _] -> w298
                      tunnel: [w316 _] -> _
                      tunnel: w292 -> [w315 _]
                      tunnel: w291 -> [w314 _]
                      tunnel: w290 -> [w313 _]
                      tunnel: w289 -> [w312 _]
                      tunnel: w287 -> [w311 _]
                      tunnel: w286 -> [w310 _]
                      tunnel: w274 -> [w303 _]
                      tunnel: w273 -> [w309 _]
                      tunnel: w275 -> [w308 _]
                      tunnel: w270 -> [w307 _]
                      tunnel: w269 -> [w306 _]
                      tunnel: 2e-05 -> [w305 _]
                      tunnel: 2e-05 -> [w304 _]
                      tunnel: 0.091 -> [w302 _]
                      tunnel: [w301 _] -> w265
                      frame False {
                        # "Evaporative Cooling"
                        n73 = formula code="f100=U1/((1+(time/tau))**beta);\nPmod=f100*10**-6*3.14159*wx*wy*kb/(2*alpha);\noffset=3;\nx=abs(Pmod/Pmax);\nV=-65.186*x**5+176.18*x**4-182.5*x**3+91.63*x**2-27.285*x+7.3877+offset;"("U1"=w303, "time"=w310, "t1"=w315, "c2"=w309, "tau"=w308, "fmod"=w314, "A2"=w313, "beta"=w311, "g2"=w312, "kb"=w306, "alpha"=w307, "wx"=w304, "wy"=w305, "Pmax"=w302) -> ("f100"=w316:dbl, "time"=w317:dbl, "V"=w318:dbl, "Pmod"=w301:dbl)  [unwired: 2 out]
                      }
                      frame True {
                        n74 = stacked-sequence {
                          frame #0 {
                            n75 = One Button Dialog(message="Either the initial or the final DC value exceeds the peak to peak voltage (\"constant\") set.  Please change the values and try again.") -> ()  [unwired: 1 in, 1 out]
                          }
                          frame #1 {
                            n76 = Stop(stop? (T)=TRUE) -> ()
                          }
                        }
                      }
                    }
                    n77 = Divide(x=w272, y=w285) -> (x/y=w284:dbl)
                  }
                }
              }
              n78 = Add(x=w128, y=w126) -> (x+y=w127:dbl[])
              n79 = Build Array (concatenate)(w122, w124) -> (w123:dbl[])
              n80 = Build Array (concatenate)(w139, w127) -> (w140:dbl[])
              n81 = Build Array (concatenate)(w136, w137) -> (w138:dbl[])
              n82 = Divide(x=w125, y=1000.0) -> (x/y=w130:dbl)
              n83 = Add(x=w130, y=w126) -> (x+y=w132:dbl)
              "x+y 2" <- w132
            }
          }
        }
        n84 = Array Size(array=w87) -> (size(s)=w86:i32)
        n85 = Bundle By Name("dt"=w90, "Y"=w87) -> (w89:waveform(dbl))  [unwired: 1 in]
        n86 = Build Array (concatenate)(w87, 0) -> (w92:dbl[])
        n87 = Bundle(w88, w87) -> (w94:cluster{dbl[], dbl[]})  [unwired: 1 in]
      }
      "signal out" <- w19
      "Array" <- w29
      "Pmod Graph" <- w16
      n88 = Index Array(array=w36, index="Channel to plot") -> (element=→"Waveform on Channel to Plot":cluster{dbl[], dbl[]})
    }
    frame #1 {
      w368 = 10214 items=["High"=10192, "Low"=10214] ("idle state")
      w370 = 10280 items=["Rising"=10280, "Falling"=10171] ("edge")
      w376 = 10178 items=["Finite Samples"=10178, "Continuous Samples"=10123, "Hardware Timed Single Point"=12522] ("sample mode")
      w379 = T4 3 items=["no dialog", "OK message", "continue or stop message", "OK message + warnings", "continue/stop + warnings"] ("type of dialog (OK msg:1)")
      w380 = 10123 items=["Finite Samples"=10178, "Continuous Samples"=10123, "Hardware Timed Single Point"=12522] ("sample mode")
      # "Physical Channel"
      # "Counter Channel"
      # "sampling rate"
      # "total points"
      # "write voltage values to intermediate buffer"
      # "write waveform"
      # "device 7:\n6229 board"
      n89 = case shown="15" w336 {
        tunnel: [_ refnum<k21> "NI6229 AO 00" ("global virtual channels") refnum<k21> "NI6229 AO 01" ("global virtual channels") refnum<k21> "NI6229 AO 02" refnum<k21> "NI6229 AO 03" refnum<k21> "NI6229 AO 00:01" refnum<k21> "NI6229 AO 00, NI6229 AO 02" refnum<k21> "NI6229 AO 00, NI6229 AO 03" refnum<k21> "NI6229 AO 01:02" refnum<k21> "NI6229 AO 01, NI6229 AO 03" refnum<k21> "NI6229 AO 02:03" refnum<k21> "NI6229 AO 00:02" refnum<k21> "NI6229 AO 00:01, NI6229 AO 03" refnum<k21> "NI6229 AO 00, NI6229 AO 02:03" refnum<k21> "NI6229 AO 01:03" refnum<k21> "NI6229 AO 00:03"] -> w337
        frame 0, Default {
          # "Program no channels"
        }
        frame 1 {
        }
        frame 2 {
        }
        frame 3 {
        }
        frame 4 {
        }
        frame 5 {
        }
        frame 6 {
        }
        frame 7 {
        }
        frame 8 {
        }
        frame 9 {
        }
        frame 10 {
        }
        frame 11 {
        }
        frame 12 {
        }
        frame 13 {
        }
        frame 14 {
        }
        frame 15 {
        }
      }
      n90 = property class="DAQmx Device"("Active Device"=tag "Dev7") -> ("Identification:Product Type"=w341:string)  [unwired: 2 in, 2 out]
      n91 = Equal?(x=w341, y="PCI-6229") -> (x = y?=w383:bool)
      n92 = case shown="True" w383 {
        tunnel: [w411 "PCI-6229 OK"] -> w382
        tunnel: "error in" -> [w412 w413]
        tunnel: [w410 w413] -> w344
        frame False {
          w411 = "PCI-6221 not found."
          n93 = Unbundle(w412) -> ()  [unwired: 3 out]
          n94 = Bundle(cluster=w412, "source"=w411) -> (w410:errorcluster)  [unwired: 2 in]
        }
        frame True {
        }
      }
      "6229 Status" <- w382
      n95 = case shown="True" "Case Constant\n(See Context Help) 3" {
        tunnel: w347 -> [_ w404]
        tunnel: w346 -> [_ w403]
        tunnel: w344 -> [w400 w402]
        tunnel: [w400 w402] -> w343
        tunnel: [_ w401] -> _
        frame False {
        }
        frame True {
          # "Clears tasks _before_ writing new waveform.\nError is not hooked up so that program will finish\nrunning either way."
          n96 = call <vilib>:"DAQmx Stop Task.vi"("task/channels in"=w403) -> ("task out"=w408:refnum<k21>, "error out"=w409:errorcluster)  [unwired: 13 in]
          n97 = call <vilib>:"DAQmx Clear Task.vi"("task in"=w408, "error in"=w409) -> ("error out"=w405:errorcluster)  [unwired: 13 in]
          n98 = call <vilib>:"DAQmx Stop Task.vi"("task/channels in"=w404, "error in"=w405) -> ("task out"=w406:refnum<k21>, "error out"=w407:errorcluster)  [unwired: 12 in]
          n99 = call <vilib>:"DAQmx Clear Task.vi"("task in"=w406, "error in"=w407) -> ("error out"=w401:errorcluster)  [unwired: 13 in]
        }
      }
      n100 = call <vilib>:"DAQmx Create Task.vi"("new task name"="Lattice Loading", "auto cleanup"=FALSE, "global virtual channels"=w337, "error in"=w343) -> ("task out"=w359:refnum<k21>, "error out"=w360:errorcluster)  [unwired: 10 in]
      n101 = call-poly <vilib>:"DAQmx Timing.vi"("task/channels in"=w359, "sample mode"=w380, "rate"=w361, "source"=tag "/Dev7/Ctr0InternalOutput", "error in"=w360) -> ("task out"=w364:refnum<k21>, "error out"=w363:errorcluster)  [unwired: 9 in]
      n102 = call-poly <vilib>:"DAQmx Write.vi"("task/channels in"=w364, "data"=w335, "timeout"=10.0, "error in"=w363) -> ("task out"=w365:refnum<k21>, "number of samples written per channel"=→"number of samples written per channel":u32, "error out"=w350:errorcluster)  [unwired: 9 in]
      n103 = call <vilib>:"DAQmx Create Task.vi"("new task name"="Lattice Counter Output", "auto cleanup"=FALSE, "error in"=w350) -> ("task out"=w351:refnum<k21>, "error out"=w349:errorcluster)  [unwired: 11 in]
      n104 = call-poly <vilib>:"DAQmx Create Virtual Channel.vi"("task in"=w351, "frequency"=w361, "counter"=tag "Dev7/ctr0", "error in"=w349, "idle state"=w368) -> ("task out"=w358:refnum<k21>, "error out"=w377:errorcluster)  [unwired: 9 in]
      n105 = call-poly <vilib>:"DAQmx Timing.vi"("task/channels in"=w358, "sample mode"=w376, "samples per channel"=w334, "error in"=w377) -> ("task out"=w372:refnum<k21>, "error out"=w375:errorcluster)  [unwired: 10 in]
      n106 = call-poly <vilib>:"DAQmx Trigger.vi"("task/channels in"=w372, "source"=tag "/Dev7/PFI0", "edge"=w370, "error in"=w375) -> ("task out"=w373:refnum<k21>, "error out"=w374:errorcluster)  [unwired: 10 in]
      n107 = property class="DAQmx Trigger"(reference=w373, error in=w374, "Start:More:Retriggerable"=TRUE ("Start.Retriggerable")) -> (reference out=w371:refnum<k21>, error out=w366:errorcluster)
      n108 = call <vilib>:"DAQmx Start Task.vi"("task/channels in"=w365, "error in"=w366) -> ("task out"=→"6229 lattice loading task out":refnum<k21>, "error out"=w367:errorcluster)  [unwired: 12 in]
      n109 = call <vilib>:"DAQmx Start Task.vi"("task/channels in"=w371, "error in"=w367) -> ("task out"=→"6229 counter task out":refnum<k21>, "error out"=w338:errorcluster)  [unwired: 12 in]
      n110 = call <vilib>:"Simple Error Handler.vi"("type of dialog (OK msg:1)"=w379, "error in (no error)"=w338) -> ("error out"=→"error out":errorcluster)  [unwired: 3 in, 4 out]
      "wvfrm size" <- w334
    }
  }
